vi "sim_test.vi"() -> ()   [LabVIEW 2014]
uses:
  <vilib>/userdefined/High Color/IMAQdx.ctl
  <vilib>/vision/driver/NI_Vision_Acquisition_Software.lvlib
  <resource>/objmgr/imaqdx.rc
panel:
  out "length 2":i32
  out "length":i32
  out "x = y?":bool
  out "size(s)":i32
  in  "bytes per packet":i32
  out "Image 2":T1(plugin-control)
  in  "Type of Flatten (Image and Vision Info)":i32(ring)=1 items=["Image", "Image and Vision Info", "Reference to Image"]
  in  "Compression (None)":i32(ring) items=["None", "JPEG", "PACKED BINARY"]
  out "Image":T1(plugin-control)
  in  "VideoMode":u32
  in  "Session In":T2
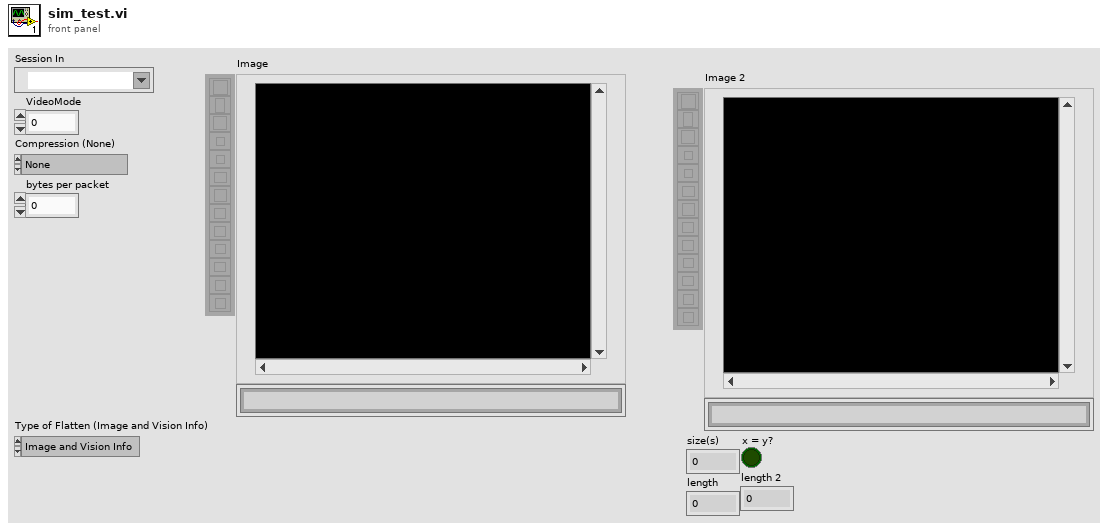
[diagram p1: front panel]
types:
  T1 = typedef "IMAQ Image.ctl" = refnum<image>
  T2 = typedef "IMAQdx.ctl" = refnum<k21>
  T3 = cluster{"pkt_idx":u32, "pkt_size":u32, "payload":string}[]
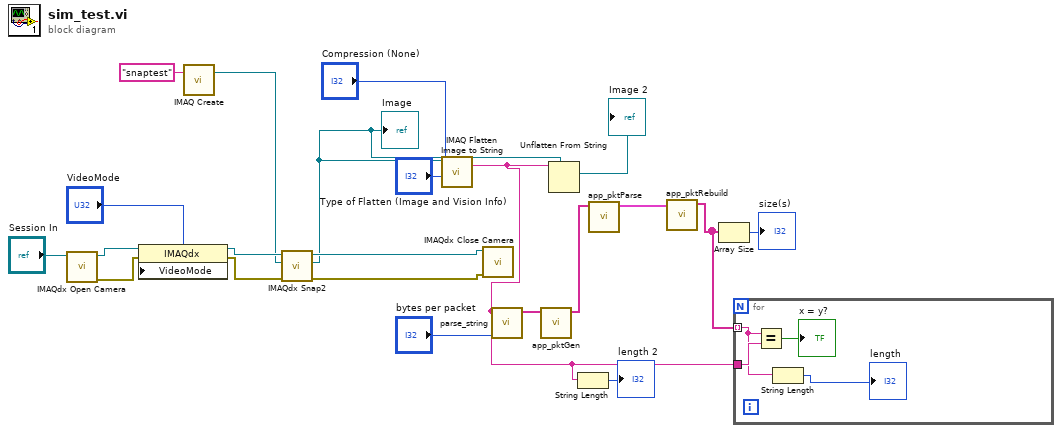
[diagram p0: block diagram]
diagram:
  n1 = call <vilib>:"IMAQdx Open Camera.vi"("Session In"="Session In") -> ("error out"=w21:errorcluster, "Session Out"=w22:T2)  [unwired: 9 in]
  n2 = property class="IMAQdx"(reference=w22, error in=w21, "VideoMode"="VideoMode") -> (reference out=w17:T2, error out=w16:errorcluster)
  n3 = call "IMAQ Create"("Image Name"="snaptest") -> ("New Image"=w15:T1)  [unwired: 4 in, 1 out]
  n4 = call <vilib>:"IMAQdx Snap2.vi"("error in"=w16, "Image In"=w15, "Session In"=w17) -> ("error out"=w13:errorcluster, "Image Out"=w10:T1, "Session Out"=w14:T2)  [unwired: 6 in]
  "Image" <- w10
  n5 = call "IMAQ Flatten Image to String"("Type of Flatten (Image and Vision Info)"="Type of Flatten (Image and Vision Info)", "Compression (None)"="Compression (None)", "Image"=w10) -> ("Data String"=w2:string)  [unwired: 7 in, 1 out]
  n6 = call <vilib>:"IMAQdx Close Camera.vi"("error in"=w13, "Session In"=w14) -> ()  [unwired: 9 in, 1 out]
  n7 = call "parse_string.vi"("bytes per packet"="bytes per packet", "original content"=w2) -> ("appended array"=w7:string[])  [unwired: 9 in]
  n8 = call "app_pktGen.vi"("appended array"=w7) -> ("packets"=w6:string[])  [unwired: 10 in]
  n9 = Unflatten From String(type=w10, binary string=w2) -> (value=→"Image 2":T1)  [unwired: 3 in, 2 out]
  n10 = String Length(string=w2) -> (length=→"length 2":i32)
  n11 = call "app_pktParse.vi"("pkts_get"=w6) -> ("app_pkt"=w5:T3)  [unwired: 9 in, 1 out]
  n12 = call "app_pktRebuild.vi"("app_pkt"=w5) -> ("out pkts"=w3:string[])  [unwired: 10 in]
  n13 = Array Size(array=w3) -> (size(s)=→"size(s)":i32)
  n14 = for {
    tunnel: w3 -> [w24] mode=indexing
    tunnel: w2 -> [w26]
    n15 = Equal?(x=w24, y=w26) -> (x = y?=→"x = y?":bool)
    n16 = String Length(string=w24) -> (length=→"length":i32)
  }
